vi "Read_command_file.vi"() -> ()   [LabVIEW 2016]
uses:
  Instrument_Setup.vi
  Global Variables/Globale Variablen Torque.vi
  Global Variables/global.vi
panel:
  out "Array":dbl[][](array[numeric])
  out "String":string
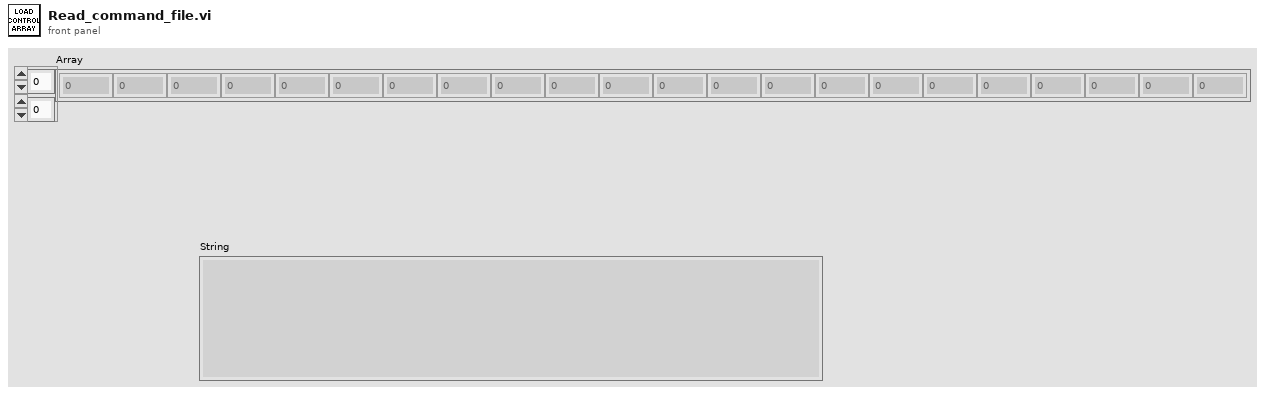
[diagram p1: front panel]
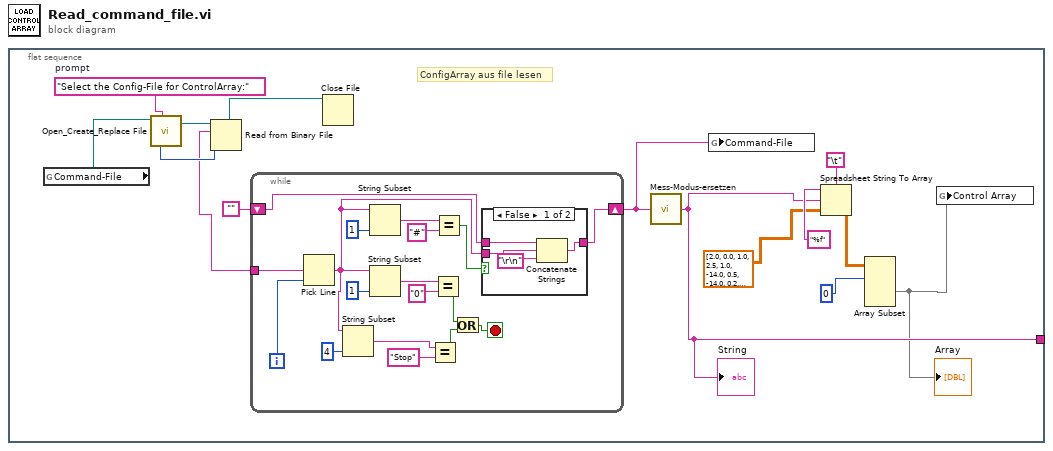
[diagram p0: block diagram]
diagram:
  n1 = flat-sequence {
    tunnel: [w3] -> _
    frame #0 {
      w14 = "Select the Config-File for ControlArray:"  # prompt
      # "ConfigArray aus file lesen"
      n2 = global read "Instrument_Setup.vi" "Command-File"() -> (w7:path)
      n3 = call <vilib>:"Open_Create_Replace File.vi"("prompt"=w14, "file path"=w7) -> ("file size (bytes)"=w13:i32, "refnum"=w15:refnum<file>)  [unwired: 6 in, 2 out]
      n4 = Read from Binary File ("Read File")(10:w13, 11:w15) -> (2:w5:string, 3:w12:refnum<file>)  [unwired: 4 in, 2 out]
      n5 = while {
        tunnel: w5 -> [w25]
        shift-right: [w28] -> w4
        shift-left: "" -> [w24]
        i -> [w33]
        stop <- w21 stop-if-true
        n6 = Pick Line(multi-line string=w25, line index=w33) -> (output string=w17:string)  [unwired: 1 in]
        n7 = String Subset(string=w17, length (rest)=4 ("Länge (Rest)")) -> (substring=w16:string)  [unwired: 1 in]
        n8 = String Subset(string=w17, length (rest)=1 ("Länge (Rest)")) -> (substring=w31:string)  [unwired: 1 in]
        n9 = String Subset(string=w17, length (rest)=1 ("Länge (Rest)")) -> (substring=w23:string)  [unwired: 1 in]
        n10 = Equal?(x=w16, y="Stop") -> (x = y?=w19:bool)
        n11 = Equal?(x=w23, y="0") -> (x = y?=w20:bool)
        n12 = Equal?(x=w31, y="#") -> (x = y?=w29:bool)
        n13 = Or(x=w20, y=w19) -> (x .or. y?=w21:bool)
        n14 = case shown="False" w29 {
          tunnel: w24 -> [w35 w38]
          tunnel: [w37 w38] -> w28
          tunnel: w17 -> [w34 _]
          frame False {
            n15 = Concatenate Strings(w35, w34, "\r\n") -> (w37:string)
          }
          frame True {
          }
        }
      }
      n16 = Close File(refnum=w12) -> ()  [unwired: 1 in, 2 out]
      n17 = call "Mess-Modus-ersetzen.vi"("Eingangs-String"=w4) -> ("Ergebnis-String"=w3:string)
      "String" <- w3
      n18 = global write "Globale Variablen Torque.vi" "Command-File"(w4) -> ()
      n19 = Spreadsheet String To Array(delimiter (Tab)="\t", format string="%f", spreadsheet string=w3, array type (2D Dbl)=dbl[][] [[2.0, 0.0, 1.0, 2.5, 1.0, -14.0, 0.5, -14.0, 0.2, 19.0, 13.0, 0.0, 0.0, 0.0, 280.0, 0.0, 0.0, 45.0, 0.0, 0.0001, 22.08, 1e-05], [0.0, 0.0, 0.0, 0.0, 0.0, 0.0, 0.0, 0.0, 0.2, 0.0, 0.0, 0.0, 0.0, 0.0, 0.0, 0.0, 0.0, 0.0, 0.0, 0.0, 0.0, 0.0]] ("Array 3")) -> (array=w9:dbl[][])
      n20 = Array Subset(array=w9, index (row)=0) -> (w2:dbl[][])  [unwired: 3 in]
      "Array" <- w2
      n21 = global write "global.vi" "Control Array"(w2) -> ()
    }
  }
